vi "ALONE_BLUEFORS.vi"(6 "Refresco(s)":dbl=5.0 caption="Elapsed Time (s)" format="%.2f", 8 "error in (no error)":errorcluster) -> (0 "Error Out":errorcluster)   [LabVIEW 2017]
uses:
  WEB Readings/Temperaturas Bluefors.ctl
  <vilib>/Analysis/baseanly.llb/Mean (DBL).vi
  cRIO_ZNB_AMI_GLOBALES.vi
  <vilib>/gmath/NI_Gmath.lvlib
  <vilib>/Analysis/NI_AALBase.lvlib
panel:
  out "Ch":u8
  in  "Radio Buttons":enum32{"50K", "4K", "Mag", "Still", "MXC"}(radio)
  out "T_MXC":dbl format="%.2f"
  out "T_Still":dbl format="%.2f"
  out "T_Mag":dbl format="%.2f"
  out "T_4K":dbl format="%.2f"
  out "BLUEFORS":T1 {"Canal 8" format="%.3f"; "Canal 7" format="%.3f"; "Canal 6" format="%.3f"; "Canal 5" format="%.3f"; "Canal 4" format="%.3f"; "Canal 3" format="%.3f"; "Canal 2" format="%.3f"; "Canal 1" format="%.3f"}
  in  "url":string="http://192.168.0.101:5001/channel/measurement/latest"
  in  "Web(T)":bool=TRUE
  out "New":bool
  out "String":string
  out "Temp Chart":dbl(graph)
  out "Array":dbl[](array[numeric])
  in  "q":i32=5 caption="Puntos, q" format="%#.0f"
  out "T Stable (T:yes)":bool caption="Estable"
  in  "sd max, %":dbl=5.0 caption="Desviacion max, %" format="%.1f"
  in  "Error max (K)":dbl=1.0 caption="Error" format="%.3f"
  out "Temperature Status":i32(ring) items=["TemperatureUnknown", "Stable", "Tracking", "Near"]
  out "Num 1":i32
  out "T_50K":dbl format="%.2f"
  out "Error":bool
  out "Date":string caption="asd"
  out "Time":string
  out "Refresh":bool
  in  "stop":bool
  # "Controlador BLUEFORS"
  # "STATUS"
  # "SETTINGS"
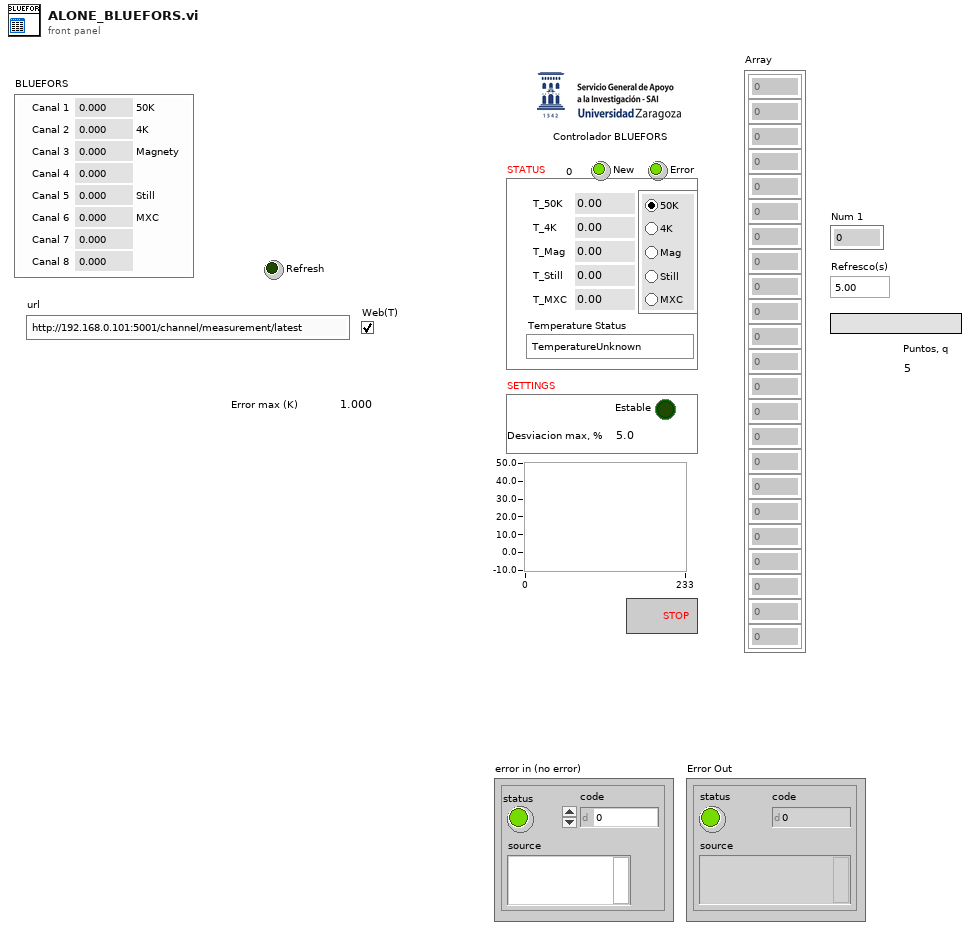
[diagram p1: front panel]
types:
  T1 = typedef "Temperaturas Bluefors.ctl" = cluster{"Canal 1":dbl, "Canal 2":dbl, "Canal 3":dbl, "Canal 4":dbl, "Canal 5":dbl, "Canal 6":dbl, "Canal 7":dbl, "Canal 8":dbl}
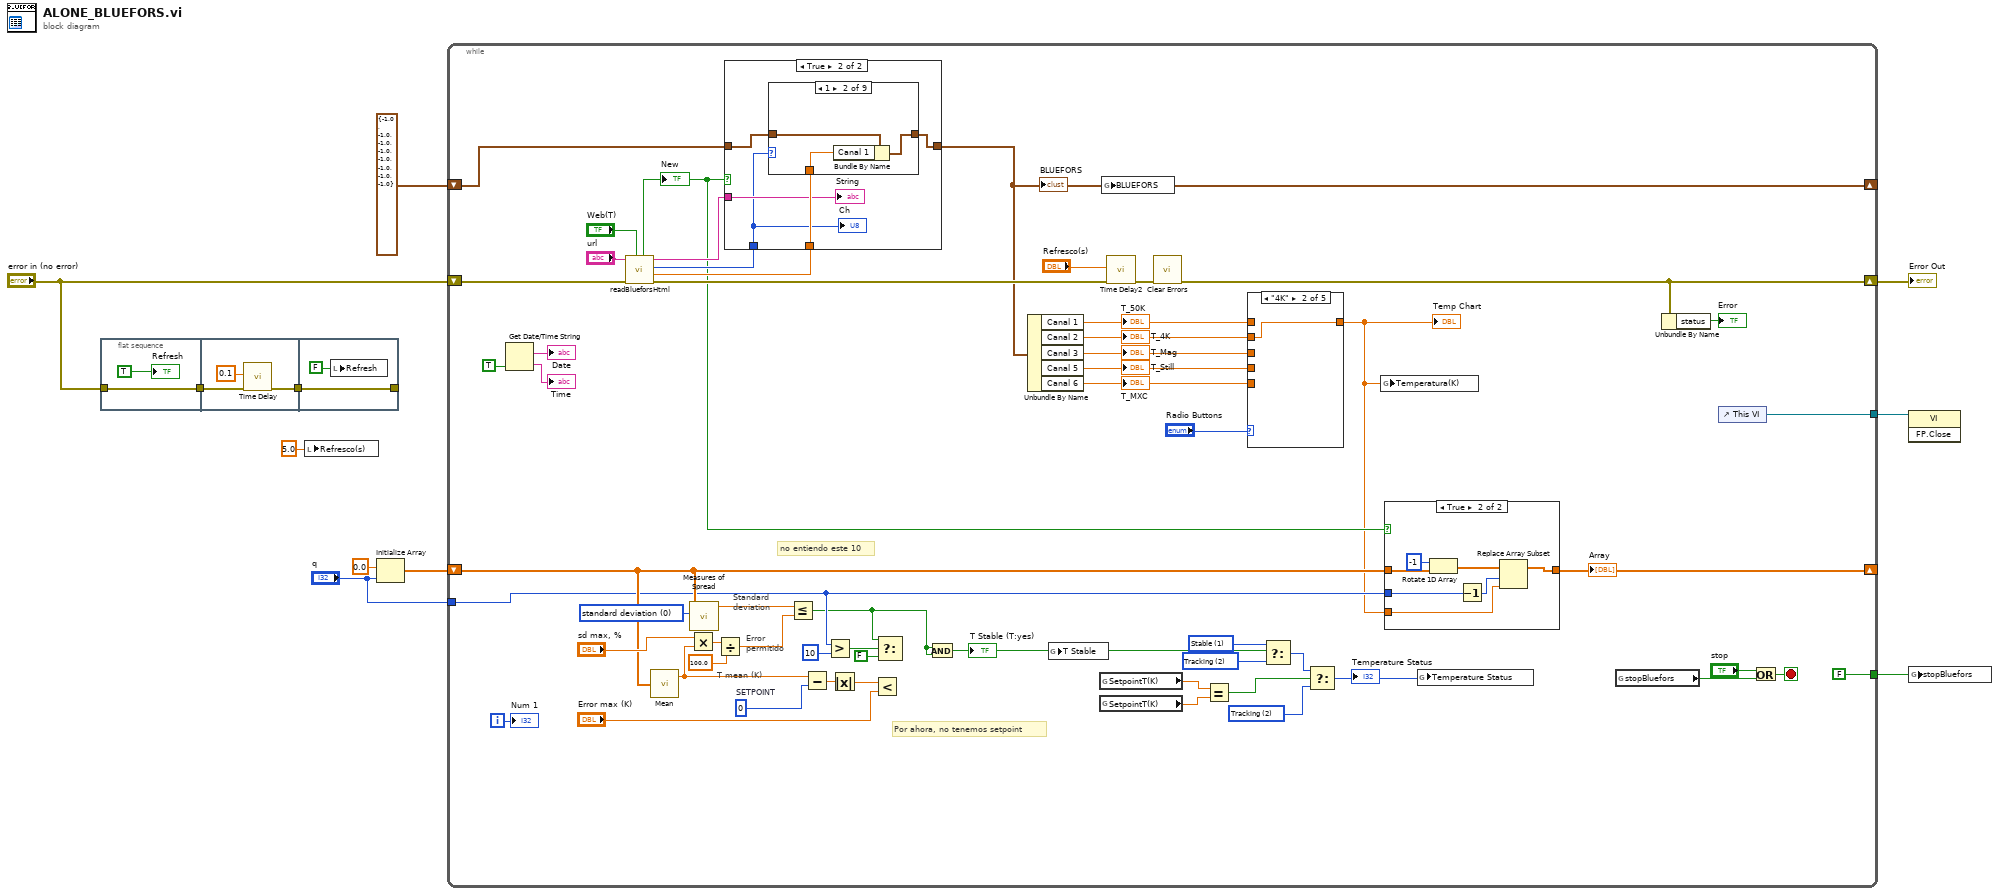
[diagram p0: block diagram]
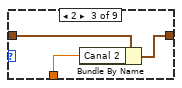
[diagram p9: hidden frame]
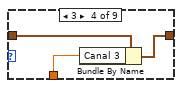
[diagram p10: hidden frame]
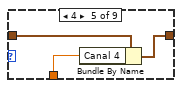
[diagram p11: hidden frame]
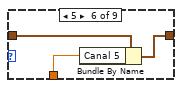
[diagram p12: hidden frame]
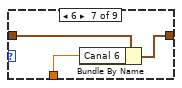
[diagram p13: hidden frame]
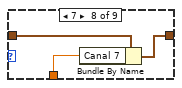
[diagram p14: hidden frame]
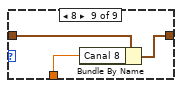
[diagram p15: hidden frame]
diagram:
  n1 = flat-sequence {
    tunnel: "error in (no error)" -> [w13]
    tunnel: [w13] -> w4
    tunnel: w4 -> [w15]
    tunnel: [w14] -> w3
    tunnel: [w17] -> _
    tunnel: w3 -> [w17]
    frame #0 {
      "Refresh" <- TRUE ("Refresh")
    }
    frame #1 {
      n2 = call "Time Delay"("error in (no error)"=w15, "Delay Time (s)"=0.1) -> ("error out"=w14:errorcluster)  [unwired: 9 in]
    }
    frame #2 {
      n3 = local write "Refresh"(FALSE ("Refresh")) -> ()
    }
  }
  n4 = local write "Refresco(s)"(5.0 ("Refresco(s)")) -> ()
  n5 = Initialize Array(0.0 ("element"), "q") -> (w8:dbl[])
  n6 = while {
    tunnel: [FALSE ("stop")] -> w10
    tunnel: [w69] -> w11
    tunnel: "q" -> [w40]
    shift-right: [w43] -> _
    shift-left: w8 -> [w44]
    shift-right: [w30] -> _
    shift-left: T1 {"Canal 1"=-1.0, "Canal 2"=-1.0, "Canal 3"=-1.0, "Canal 4"=-1.0, "Canal 5"=-1.0, "Canal 6"=-1.0, "Canal 7"=-1.0, "Canal 8"=-1.0} ("BLUEFORS") -> [w32]
    shift-right: [w24] -> w5
    shift-left: "error in (no error)" -> [w31]
    i -> [w66]
    stop <- w73 stop-if-true
    w42 = 0  # SETPOINT
    w51 = 0 items=["standard deviation", "range", "mean absolute deviation", "interquartile range"] ("type")
    w60 = 2 items=["TemperatureUnknown", "Stable", "Tracking", "Near"] ("Temperature Status")
    w59 = 2 items=["TemperatureUnknown", "Stable", "Tracking", "Near"] ("Temperature Status")
    w58 = 1 items=["TemperatureUnknown", "Stable", "Tracking", "Near"] ("Temperature Status")
    # "Por ahora, no tenemos setpoint"
    # "no entiendo este 10"
    # "Error\npermitido"
    # "Standard\ndeviation"
    # "T mean (K)"
    n7 = Get Date/Time String(want seconds? (F)=TRUE) -> (date string=→"Date":string, time string=→"Time":string)  [unwired: 2 in]
    n8 = call "readBlueforsHtml.vi"("Web(T)"="Web(T)", "Error In"=w31, "url"="url") -> ("Error Out"=w33:errorcluster, "temperatura"=w36:dbl, "chan_nr"=w35:i32, "date/time string"=w39:string, "datoNuevo?"=w22:bool)  [unwired: 3 in, 1 out]
    "New" <- w22
    n9 = call-poly <vilib>:"Mean.vi"("X"=w44) -> ("mean"=w56:dbl)  [unwired: 1 out]
    n10 = Multiply(x="sd max, %", y=w56) -> (x*y=w47:dbl)
    n11 = call <vilib>:"Measures of Spread.vi"("type"=w51, "x array"=w44) -> ("spread value"=w45:dbl)  [unwired: 8 in, 1 out]
    n12 = Divide(x=w47, y=100.0) -> (x/y=w48:dbl)
    n13 = case shown="True" w22 {
      tunnel: w32 -> [w89 w94]
      tunnel: [w89 w93] -> w30
      tunnel: w35 -> [_ w90]
      tunnel: w36 -> [_ w92]
      tunnel: w39 -> [_ w91]
      frame False {
      }
      frame True {
        n14 = case shown="1" w90 {
          tunnel: w94 -> [w95 w98 w101 w104 w107 w110 w113 w116 w119]
          tunnel: [w95 w97 w100 w103 w106 w109 w112 w115 w118] -> w93
          tunnel: w92 -> [_ w96 w99 w102 w105 w108 w111 w114 w117]
          frame 0, Default {
          }
          frame 1 {
            n15 = Bundle By Name(cluster=w98, "Canal 1"=w96) -> (w97:T1)
          }
          frame 2 {
            n16 = Bundle By Name(cluster=w101, "Canal 2"=w99) -> (w100:T1)
          }
          frame 3 {
            n17 = Bundle By Name(cluster=w104, "Canal 3"=w102) -> (w103:T1)
          }
          frame 4 {
            n18 = Bundle By Name(cluster=w107, "Canal 4"=w105) -> (w106:T1)
          }
          frame 5 {
            n19 = Bundle By Name(cluster=w110, "Canal 5"=w108) -> (w109:T1)
          }
          frame 6 {
            n20 = Bundle By Name(cluster=w113, "Canal 6"=w111) -> (w112:T1)
          }
          frame 7 {
            n21 = Bundle By Name(cluster=w116, "Canal 7"=w114) -> (w115:T1)
          }
          frame 8 {
            n22 = Bundle By Name(cluster=w119, "Canal 8"=w117) -> (w118:T1)
          }
        }
        "String" <- w91
        "Ch" <- w90
      }
    }
    "BLUEFORS" <- w30
    n23 = Less Or Equal?(x=w45, y=w48) -> (x <= y?=w20:bool)
    n24 = Subtract(x=w56, y=w42) -> (x-y=w49:dbl)
    n25 = Greater?(x=w40, y=10) -> (0:w46:bool)
    n26 = Absolute Value(x=w49) -> (abs(x)=w50:dbl)
    n27 = Less?(x=w50, y="Error max (K)") -> ()  [unwired: 1 out]
    n28 = Select(t=w20, s=w46, f=FALSE ("TdownStable (T:yes)")) -> ()  [unwired: 1 out]
    n29 = And(x=w20, y=w20) -> (x .and. y?=w41:bool)
    "T Stable (T:yes)" <- w41
    n30 = Unbundle By Name(w30) -> ("Canal 1"=w21:dbl, "Canal 2"=w28:dbl, "Canal 3"=w27:dbl, "Canal 5"=w26:dbl, "Canal 6"=w25:dbl)
    "T_50K" <- w21
    "T_4K" <- w28
    "T_Mag" <- w27
    "T_Still" <- w26
    "T_MXC" <- w25
    n31 = global write "cRIO_ZNB_AMI_GLOBALES.vi" "T Stable"(w41) -> ()
    n32 = global read "cRIO_ZNB_AMI_GLOBALES.vi" "SetpointT(K)"() -> (w65:dbl)
    n33 = global read "cRIO_ZNB_AMI_GLOBALES.vi" "SetpointT(K)"() -> (w64:dbl)
    n34 = global write "cRIO_ZNB_AMI_GLOBALES.vi" "BLUEFORS"(w30) -> ()
    n35 = call "Time Delay2"("error in (no error)"=w33, "Delay Time (s)"="Refresco(s)") -> ("error out"=w38:errorcluster)  [unwired: 9 in]
    n36 = call <vilib>:"Clear Errors.vi"("error in (no error)"=w38) -> ("error out"=w24:errorcluster)  [unwired: 5 in, 1 out]
    n37 = Equal?(x=w65, y=w64) -> (x = y?=w63:bool)
    n38 = case shown="\"4K\"" "Radio Buttons" {
      tunnel: w21 -> [w84 _ _ _ _]
      tunnel: [w84 w85 w86 w87 w88] -> w19
      tunnel: w28 -> [_ w85 _ _ _]
      tunnel: w27 -> [_ _ w86 _ _]
      tunnel: w26 -> [_ _ _ w87 _]
      tunnel: w25 -> [_ _ _ _ w88]
      frame "50K", Default {
      }
      frame "4K" {
      }
      frame "Mag" {
      }
      frame "Still" {
      }
      frame "MXC" {
      }
    }
    "Temp Chart" <- w19
    n39 = Select(t=w58, s=w41, f=w59) -> (s? t:f=w62:i32)
    n40 = Select(t=w62, s=w63, f=w60) -> (s? t:f=w61:i32)
    "Temperature Status" <- w61
    n41 = global write "cRIO_ZNB_AMI_GLOBALES.vi" "Temperatura(K)"(w19) -> ()
    n42 = case shown="True" w22 {
      tunnel: w44 -> [w76 w80]
      tunnel: [w76 w79] -> w43
      tunnel: w40 -> [_ w78]
      tunnel: w19 -> [_ w77]
      frame False {
      }
      frame True {
        n43 = Rotate 1D Array(1:w80, 2:-1 ("n")) -> (0:w82:dbl[])
        n44 = Decrement(x=w78) -> (x-1=w81:i32)
        n45 = Replace Array Subset(array=w82, new element=w77, index=w81) -> (w79:dbl[])
      }
    }
    "Array" <- w43
    n46 = global write "cRIO_ZNB_AMI_GLOBALES.vi" "Temperature Status"(w61) -> ()
    n47 = global read "cRIO_ZNB_AMI_GLOBALES.vi" "stopBluefors"() -> (w68:bool)
    n48 = Unbundle By Name(w24) -> ("status"=→"Error":bool)
    n49 = control-ref of="This VI"() -> (w69:refnum<vi>)
    n50 = Or(x="stop", y=w68) -> (x .or. y?=w73:bool)
    "Num 1" <- w66
  }
  "Error Out" <- w5
  n51 = invoke class="VI" method="FP.Close"(reference=w11) -> ()  [unwired: 2 in, 3 out]
  n52 = global write "cRIO_ZNB_AMI_GLOBALES.vi" "stopBluefors"(w10) -> ()
